vi "SbigExpose.vi"(2 "Time":u32, 3 "Sbig":string="PI1-SHUTTER", 7 "Window":T1, 9 "error in (no error)":errorcluster) -> (0 "Sbig out":string="PI1-SHUTTER", 6 "error out":errorcluster)   [LabVIEW 2009]
uses:
  Controls/SbigCommand.ctl
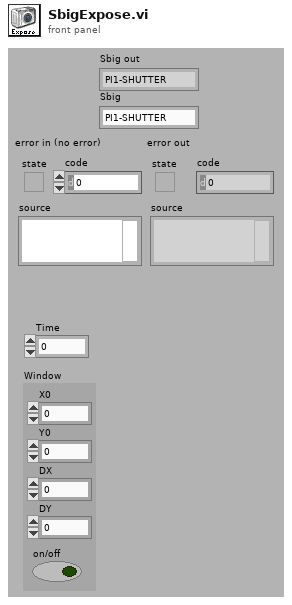
[diagram p1: front panel]
types:
  T1 = cluster{"X0":u16, "Y0":u16, "DX":u16, "DY":u16, "on/off":bool}
  T2 = typedef "SbigCommand.ctl" = cluster{"Sbig":string, "Command":enum16{"EXPOSE", "SET TEMP", "SET MISC", "QUIT"}, "Time":u32, "Window":cluster{"X0":u16, "Y0":u16, "DX":u16, "DY":u16, "on/off":bool}, "Temp":cluster{"Regulation":u16, "Auto Freeze":u16, "CCD Set Point":dbl}, "Misc":cluster{"Fan":u16, "Shutter":u16, "Led":u16}}
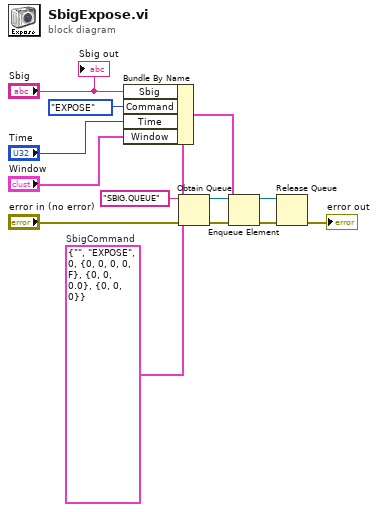
[diagram p0: block diagram]
diagram:
  w11 = T2 {"Sbig"="", "Command"=enum."EXPOSE", "Time"=0, "Window"={"X0"=0, "Y0"=0, "DX"=0, "DY"=0, "on/off"=FALSE}, "Temp"={"Regulation"=0, "Auto Freeze"=0, "CCD Set Point"=0.0}, "Misc"={"Fan"=0, "Shutter"=0, "Led"=0}}  # SbigCommand
  n1 = Bundle By Name(cluster=w11, "Sbig"="Sbig", "Command"=enum16{"EXPOSE", "SET TEMP", "SET MISC", "QUIT"}."EXPOSE", "Time"="Time", "Window"="Window") -> (w10:T2)
  n2 = Obtain Queue(name (unnamed)="SBIG.QUEUE" ("nom (aucun)"), element data type=w11, error in (no error)="error in (no error)") -> (queue out=w13:refnum<queue>, error out=w12:errorcluster)  [unwired: 2 in, 1 out]
  n3 = Enqueue Element(queue=w13, element=w10, error in (no error)=w12) -> (queue out=w8:refnum<queue>, error out=w9:errorcluster)  [unwired: 2 out]
  n4 = Release Queue(queue=w8, error in (no error)=w9) -> (error out=→"error out":errorcluster)  [unwired: 3 out]
  "Sbig out" <- "Sbig"
